vi "Test MCP4725 1.vi"() -> ()   [LabVIEW 2014]
uses:
  <vilib>/LabVIEW Universal Transcriptor/MCP4725/MCP4725.lvclass
  <vilib>/LabVIEW Universal Transcriptor/LabVIEW for Arduino Math Library/Arduino Math.lvlib
panel:
  out "MCP4725 out":refnum<class "MCP4725.lvclass">
  out "error out":errorcluster
  out "Error Out":errorcluster
  in  "Error In":errorcluster
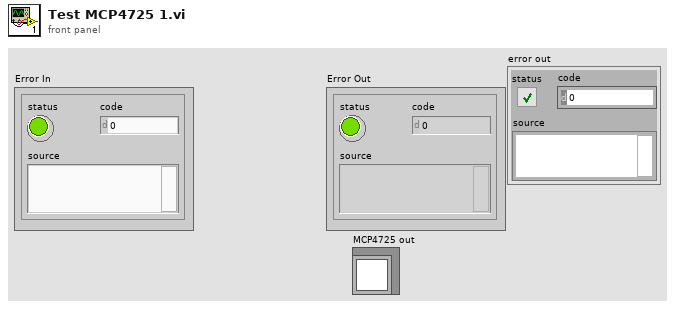
[diagram p1: front panel]
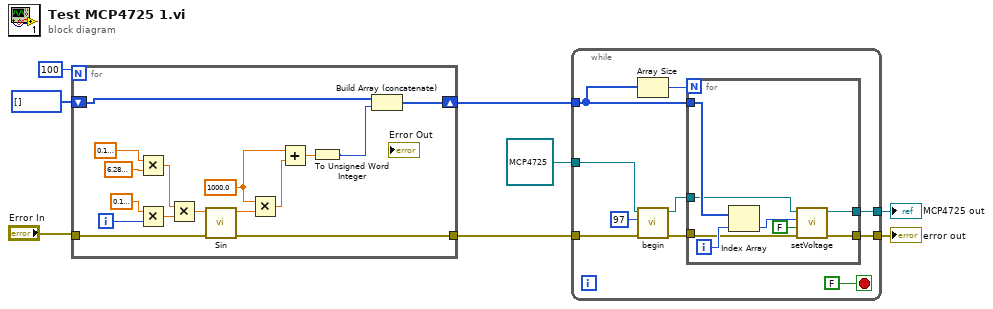
[diagram p0: block diagram]
diagram:
  n1 = for {
    N: 100 -> [_]
    tunnel: "Error In" -> [w12]
    tunnel: [w11] -> w5
    shift-right: [w13] -> w3
    shift-left: u16[] [] -> [w14]
    i -> [w21]
    w15 = sgl 1000.0 ("x")
    n2 = Multiply(x=sgl 0.1, y=sgl 6.28 ("x")) -> (x*y=w22:sgl)
    n3 = Multiply(x=sgl 0.1, y=w21) -> (x*y=w19:sgl)
    n4 = Multiply(x=w22, y=w19) -> (x*y=w18:sgl)
    n5 = call <vilib>:"Sin.vi"("Error In"=w12, "x"=w18) -> ("Error Out"=w11:errorcluster, "sin(x)"=w17:sgl)  [unwired: 8 in]
    n6 = Multiply(x=w15, y=w17) -> (x*y=w16:sgl)
    n7 = Add(x=w15, y=w16) -> (x+y=w10:sgl)
    n8 = To Unsigned Word Integer(number=w10) -> (unsigned 16bit integer=w9:u16)
    n9 = Build Array (concatenate)(w14, w9) -> (w13:u16[])
  }
  n10 = while {
    tunnel: w5 -> [w34]
    tunnel: refnum<class "MCP4725.lvclass"> refnum ("MCP4725 in") -> [w32]
    tunnel: w3 -> [w30]
    tunnel: [w27] -> w1
    tunnel: [w26] -> w2
    stop <- FALSE stop-if-true
    n11 = Array Size(array=w30) -> (size(s)=w31:i32)
    n12 = call <vilib>:"begin.vi"("error in (no error)"=w34, "I2C addr"=u8 97, "MCP4725 in"=w32) -> ("error out"=w29:errorcluster, "MCP4725 out"=w28:refnum<class "MCP4725.lvclass">)  [unwired: 7 in]
    n13 = for {
      N: w31 -> [_]
      tunnel: w30 -> [w41]
      tunnel: w29 -> [w38]
      tunnel: [w37] -> w26
      tunnel: w28 -> [w36]
      tunnel: [w35] -> w27
      i -> [w42]
      n14 = Index Array(array=w41, index=w42) -> (element=w40:u16)
      n15 = call <vilib>:"setVoltage.vi"("error in (no error)"=w38, "writeEEPROM?"=FALSE, "voltage"=w40, "MCP4725 in"=w36) -> ("error out"=w37:errorcluster, "MCP4725 out"=w35:refnum<class "MCP4725.lvclass">)  [unwired: 6 in]
    }
  }
  "error out" <- w2
  "MCP4725 out" <- w1
